vi "Remove APU Angle RTM Dependency.vi"(8 "error in (no error)":errorcluster, 9 "Menu hierarchy in":string[](array[string]), 11 "Node Ptr":u64 format="%.0x") -> (0 "error out":errorcluster, 1 "Menu hierarchy out":string[](array[string]), 3 "Action":T1)   [LabVIEW 2011, in "Engine Sim System Explorer.lvlib"]
uses:
  Engine Sim System Explorer.lvlib
  <vilib>/NI Veristand/Custom Device API/Custom Device RTM Dependency.ctl
  TypeDefs/APUComp.ctl
  Shared/Engine Simulation Global.vi
  <vilib>/NI Veristand/Custom Device API/Get Item Property (Variant).vi
  <vilib>/NI Veristand/Custom Device API/Custom Device API.lvlib
  Engine Simulation Shared.lvlib
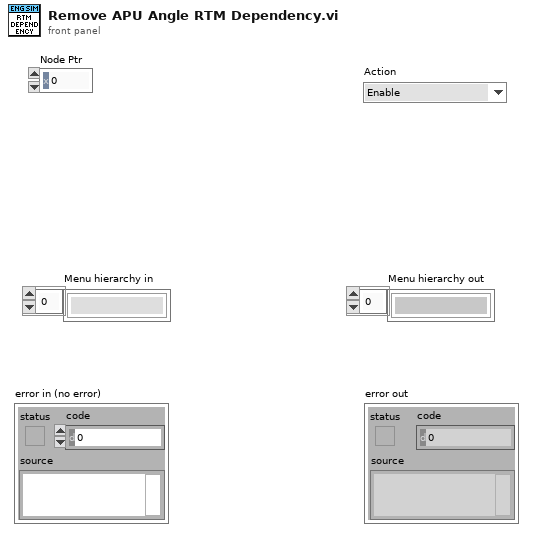
[diagram p1: front panel]
types:
  T1 = typedef "Custom Device API.lvlib/Custom Device RTM Dependency.ctl" = enum16{"Enable", "Disable", "Hide"}
  T2 = typedef "Engine Sim System Explorer.lvlib/APUComp.ctl" = cluster{"Crank Angle":bool, "Cycle Angle":bool, "Reset":bool}
  T3 = typedef "Custom Device API.lvlib/Custom Device Item Ref.ctl" = u64
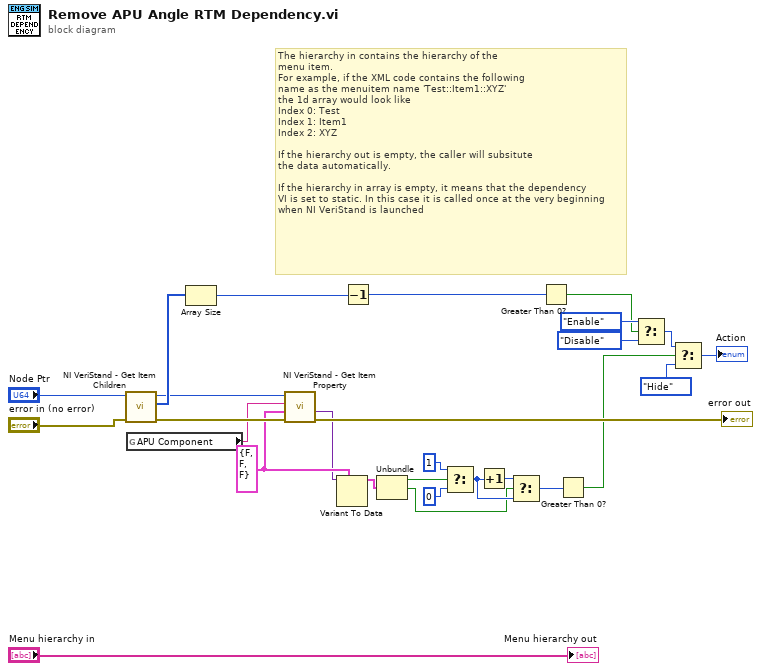
[diagram p0: block diagram]
diagram:
  w13 = T2 {"Crank Angle"=FALSE, "Cycle Angle"=FALSE, "Reset"=FALSE} ("APU Component")
  # "The hierarchy in contains the hierarchy of the\nmenu item.\nFor example, if the XML code contains the following\nname as the menuitem name 'Test::Item1::XYZ'\nthe 1d array would look like\nIndex 0: Test\nIndex 1: Item1\nIndex 2: XYZ\n\nIf the hierarchy out is empty, the caller will subsitute\nthe data automatically.\n\nIf the hierarchy in array is empty, it means that the dependency\nVI is set to static. In this case it is called once at the very beginning\nwhen NI VeriStand is launched"
  n1 = call <vilib>:"NI VeriStand - Get Item Children.vi"("error in (no error)"="error in (no error)", "Item Ref in"="Node Ptr") -> ("error out"=w25:errorcluster, "Child Refs"=w27:T3[], "Item Ref out"=w26:T3)  [unwired: 6 in, 1 out]
  n2 = global read "Engine Simulation Global.vi" "APU Component"() -> (w14:string)
  n3 = Array Size(array=w27) -> (size(s)=w3:i32)
  n4 = call-poly <vilib>:"NI VeriStand - Get Item Property.vi"("error in (no error)"=w25, "Default Value"=w13, "Property Name"=w14, "Item Ref in"=w26) -> ("error out"=→"error out":errorcluster, "Value"=w12:variant)  [unwired: 4 in, 2 out]
  n5 = Variant To Data(type=w13, Variant=w12) -> (data=w11:T2)  [unwired: 1 in, 1 out]
  n6 = Decrement(x=w3) -> (x-1=w1:i32)
  n7 = Unbundle(w11) -> ("Crank Angle"=w9:bool, "Cycle Angle"=w5:bool)  [unwired: 1 out]
  n8 = Select(t=1, s=w9, f=0) -> (s? t:f=w6:i32)
  n9 = Increment(x=w6) -> (x+1=w7:i32)
  n10 = Select(t=w7, s=w5, f=w6) -> (s? t:f=w2:i32)
  n11 = Greater Than 0?(x=w1) -> (x > 0?=w15:bool)
  n12 = Greater Than 0?(x=w2) -> (x > 0?=w4:bool)
  n13 = Select(t=Custom_Device_RTM_Dependency."Enable" ("Action"), s=w15, f=Custom_Device_RTM_Dependency."Disable") -> (s? t:f=w19:T1)
  n14 = Select(t=w19, s=w4, f=Custom_Device_RTM_Dependency."Hide" ("Action")) -> (s? t:f=→"Action":T1)
  "Menu hierarchy out" <- "Menu hierarchy in"
